vi "Start Log.vi"(8 "error in (no error)":errorcluster, 9 "Time Stamp":timestamp, 10 "Folder":path, 11 "Event Reporter Module in":refnum<class "Event Reporter Module.lvclass">) -> (0 "error out":errorcluster, 3 "Event Reporter Module out":refnum<class "Event Reporter Module.lvclass">)   [LabVIEW 2020, in "Volatus.lvlib" / "Event Reporter Module.lvclass"]
uses:
  Event Reporter Module.lvclass
  Event Reporter Module.lvclass/Event Reporter Module.ctl
  lv-cdm/CDM-Config/CDM-Config.lvlib
  lv-cdm/CDM-Config/Format.ctl
  lv-cdm/CDM-Config/Precision.ctl
  lv-cdm/CDM-Config/Format Config.ctl
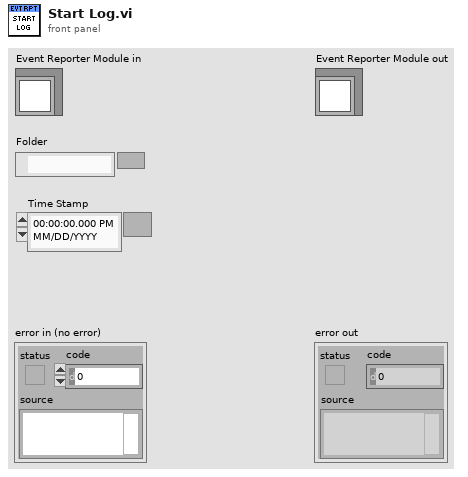
[diagram p1: front panel]
types:
  T1 = enum16{"open", "replace", "create", "open or create", "replace or create", "replace or create with confirmation"}
  T2 = typedef "CDM-Config.lvlib/Format Config.ctl" = cluster{"Format":T3, "Precision":T4}
  T3 = typedef "CDM-Config.lvlib/Format.ctl" = enum16{"Extended", "Basic"}
  T4 = typedef "CDM-Config.lvlib/Precision.ctl" = enum16{"Millisecond", "Second", "Minute", "Hour", "Day"}
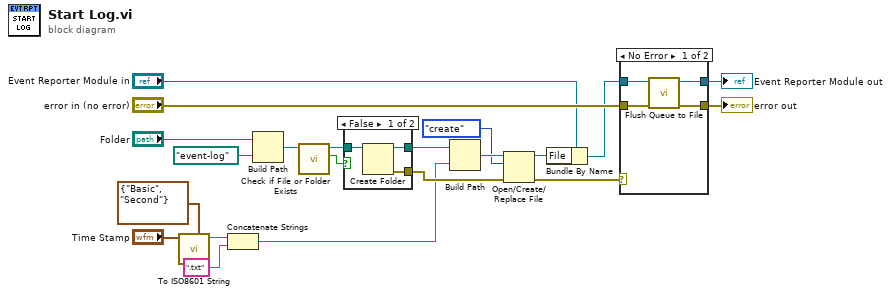
[diagram p0: block diagram]
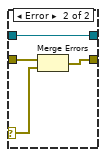
[diagram p2: hidden frame]
diagram:
  n1 = call "To ISO8601 String.vi"("Format Config"=T2 {"Format"=enum."Basic", "Precision"=enum."Second"}, "Time Stamp"="Time Stamp") -> ("ISO 8601 UTC"=w10:string)  [unwired: 9 in]
  n2 = Concatenate Strings(w10, ".txt" ("string")) -> (w8:string)
  n3 = Build Path(base path="Folder", name or relative path=path "event-log") -> (appended path=w15:path)
  n4 = call <vilib>:"Check if File or Folder Exists.vi"("path"=w15) -> ("file or folder exists?"=w14:bool, "dup path"=w13:path)  [unwired: 8 in, 1 out]
  n5 = case shown="False" w14 {
    tunnel: w13 -> [w24 w25]
    tunnel: [w23 w25] -> w7
    tunnel: [w22 _] -> w20
    frame False {
      n6 = Create Folder(path (use dialog)=w24) -> (created path=w23:path, error out=w22:errorcluster)  [unwired: 2 in, 1 out]
    }
    frame True {
    }
  }
  n7 = Build Path(base path=w7, name or relative path=w8) -> (appended path=w12:path)
  n8 = Open/Create/Replace File(file path (use dialog)=w12, error in=w20, operation (0:open)=T1."create") -> (refnum out=w6:refnum<file>, error out=w4:errorcluster)  [unwired: 3 in, 1 out]
  n9 = Bundle By Name(cluster="Event Reporter Module in", "File"=w6) -> (w2:refnum<class "Event Reporter Module.lvclass">)
  n10 = case shown="No Error" w4 {
    selector: w4 -> [_ w31]
    tunnel: [w27 w33] -> w3
    tunnel: w2 -> [w29 w33]
    tunnel: "error in (no error)" -> [w28 w32]
    tunnel: [w26 w30] -> w1
    frame No Error {
      n11 = call "Flush Queue to File.vi"("error in (no error)"=w28, "Event Reporter Module in"=w29) -> ("error out"=w26:errorcluster, "Event Reporter Module out"=w27:refnum<class "Event Reporter Module.lvclass">)  [unwired: 8 in]
    }
    frame Error {
      n12 = Merge Errors(w32, w31) -> (w30:errorcluster)
    }
  }
  "error out" <- w1
  "Event Reporter Module out" <- w3
